vi "Initialize Animation.vi"(8 "error in (no error)":errorcluster, 11 "Filled Text Fields Actor in":refnum<class "Filled Text Fields Actor.lvclass">) -> (0 "error out":errorcluster, 3 "Filled Text Fields Actor out":refnum<class "Filled Text Fields Actor.lvclass">)   [LabVIEW 2017, in "Filled Text Fields.lvlib" / "Filled Text Fields Actor.lvclass"]
uses:
  Filled Text Fields Actor.lvclass
  Filled Text Fields Actor.lvclass/Filled Text Fields Actor.ctl
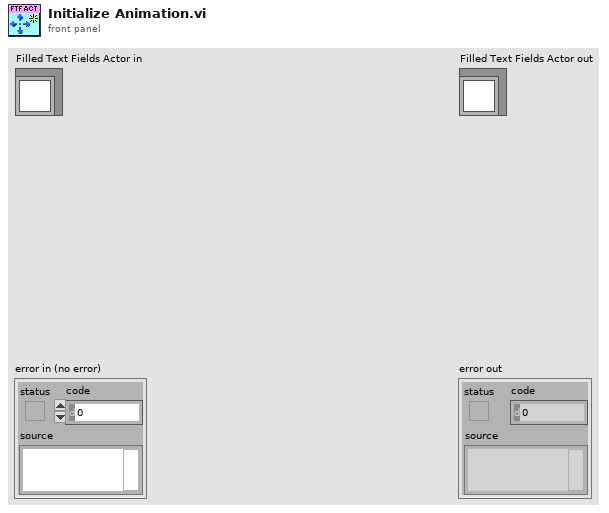
[diagram p1: front panel]
types:
  T1 = typedef "LVPositionTypeDef.ctl" = cluster{"Left":i32, "Top":i32}
  T2 = typedef "LVBoundsTypeDef.ctl" = cluster{"Width":u32, "Height":u32}
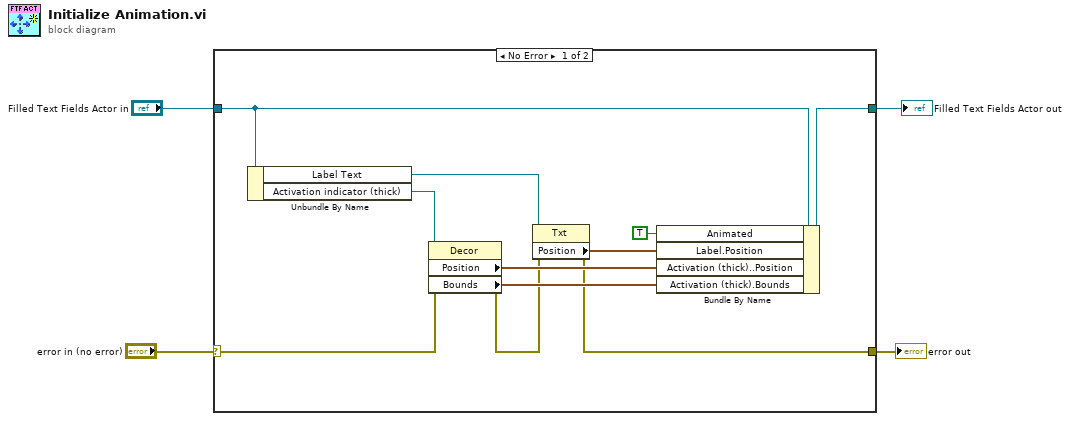
[diagram p0: block diagram]
diagram:
  n1 = case shown="No Error" "error in (no error)" {
    selector: "error in (no error)" -> [w7 w17]
    tunnel: [w6 w17] -> w3
    tunnel: [w15 w16] -> w1
    tunnel: "Filled Text Fields Actor in" -> [w14 w16]
    frame No Error {
      n2 = Unbundle By Name(w14) -> ("Label Text"=w13:refnum<vi>, "Activation indicator (thick)"=w11:refnum<vi>)
      n3 = property class="Decor"(reference=w11, error in=w7) -> (error out=w8:errorcluster, "Position"=w10:T1, "Bounds"=w9:T2)  [unwired: 1 out]
      n4 = property class="Txt"(reference=w13, error in=w8) -> (error out=w6:errorcluster, "Position"=w12:T1)  [unwired: 1 out]
      n5 = Bundle By Name(cluster=w14, "Animated"=TRUE ("Filled Text Fields.Animation.Animated"), "Label.Position"=w12, "Activation (thick)..Position"=w10, "Activation (thick).Bounds"=w9) -> (w15:refnum<class "Filled Text Fields Actor.lvclass">)
    }
    frame Error {
    }
  }
  "error out" <- w3
  "Filled Text Fields Actor out" <- w1
